vi "read Gcode.vi"(8 "error in":errorcluster, 11 "Gcode path (use dialog)":path) -> (0 "error out":errorcluster, 2 "Gcode Array":string[](array[string]), 3 "Gcode path out":path)   [LabVIEW 2020]
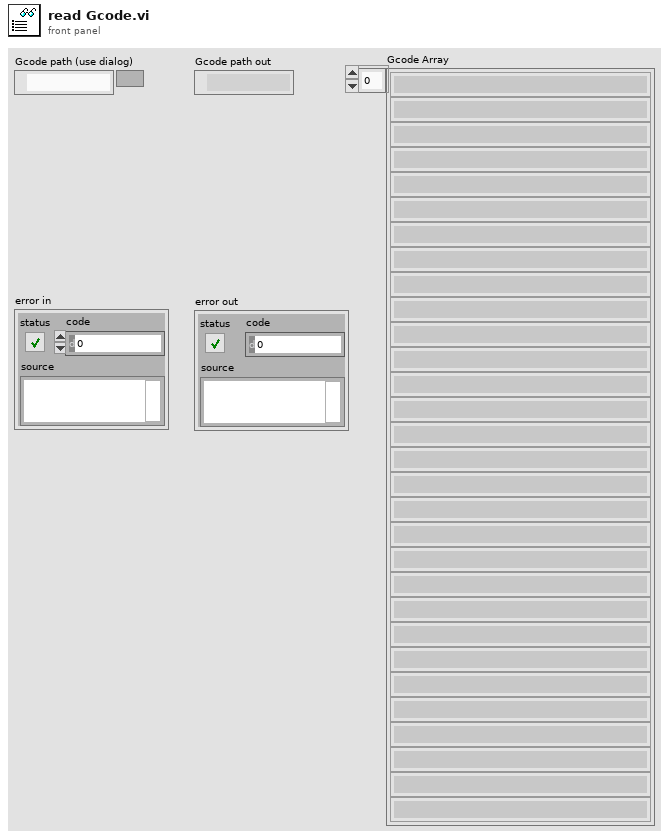
[diagram p1: front panel]
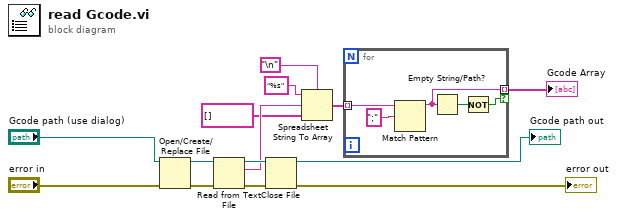
[diagram p0: block diagram]
diagram:
  n1 = Open/Create/Replace File(file path (use dialog)="Gcode path (use dialog)", error in="error in") -> (refnum out=w13:refnum<file>, error out=w12:errorcluster)  [unwired: 4 in, 1 out]
  n2 = Read from Text File(file (use dialog)=w13, error in=w12) -> (refnum out=w11:refnum<file>, text=w9:string, error out=w10:errorcluster)  [unwired: 2 in, 1 out]
  n3 = Close File(refnum=w11, error in=w10) -> (path=→"Gcode path out":path, error out=→"error out":errorcluster)
  n4 = Spreadsheet String To Array(delimiter (Tab)="\n", format string="%s", spreadsheet string=w9, array type (2D Dbl)=string[] []) -> (array=w5:string[])
  n5 = for {
    tunnel: w5 -> [w19] mode=indexing
    tunnel: [w17] -> w4 mode=indexing if=w15
    n6 = Match Pattern(string=w19, regular expression=";") -> (before substring=w17:string)  [unwired: 1 in, 3 out]
    n7 = Empty String/Path?(string/path=w17) -> (empty?=w16:bool)
    n8 = Not(x=w16) -> (.not. x?=w15:bool)
  }
  "Gcode Array" <- w4
